vi "input.vi"(8 "error in":errorcluster, 10 "input allocation":T1, 11 "LED runtime in":refnum<class "LED runtime.lvclass">) -> (0 "error out":errorcluster, 2 "input data":T1, 3 "LED runtime out":refnum<class "LED runtime.lvclass">)   [LabVIEW 2014]
doc: "Provides an interface for reading data from a module at runtime. While this interface performs no operations, a child should provide an override which may read from any open sessions, references, or interfaces."
uses:
  LED runtime.lvclass
  <vilib>/NI/Tag Bus/table/data table.ctl
  <vilib>/NI/Tag Bus/table/data table.lvlib
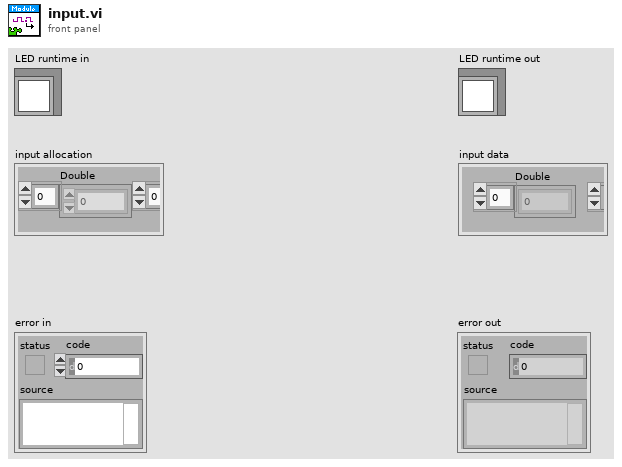
[diagram p1: front panel]
types:
  T1 = typedef "tag bus.lvlib/data table.lvlib/data table.ctl" = cluster{"Double":dbl[], "Single":sgl[], "I64":i64[], "I32":i32[], "I16":i16[], "I8":i8[], "U64":u64[], "U32":u32[], "U16":u16[], "U8":u8[], "Boolean":bool[], "String":string[], "Array of Double":cluster{"DBL Array":dbl[]}[], "Array of Single":cluster{"SGL Array":sgl[]}[], "Array of I64":cluster{"I64 Array":i64[]}[], "Array of I32":cluster{"I32 Array":i32[]}[], "Array of I16":cluster{"I16 Array":i16[]}[], "Array of I8":cluster{"I8 Array":i8[]}[], "Array of U64":cluster{"U64 Array":u64[]}[], "Array of U32":cluster{"U32 Array":u32[]}[], "Array of U16":cluster{"U16 Array":u16[]}[], "Array of U8":cluster{"U8 Array":u8[]}[], "Array of Boolean":cluster{"Boolean Array":bool[]}[], "Array of String":cluster{"String Array":string[]}[]}
  T2 = typedef "LED runtime.lvclass/input user data.ctl" = cluster{"fmwk_placeholder":i32}
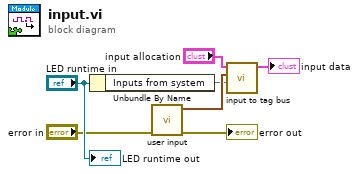
[diagram p0: block diagram]
diagram:
  n1 = Unbundle By Name("LED runtime in") -> ("Inputs from system"=w1)
  n2 = call "user input.vi"("error in"="error in") -> ("error out"=→"error out":errorcluster, "Inputs from system"=w2:T2)  [unwired: 9 in]
  n3 = call "input to tag bus.vi"("indices"=w1, "data cluster"=w2, "tag bus in"="input allocation") -> ("tag bus out"=→"input data":T1)  [unwired: 8 in]
  "LED runtime out" <- "LED runtime in"
